vi "Pins Names Read.vi"(4 "error in (no error)":errorcluster, 6 "Container State":T2, 7 "Display State In":T1) -> (0 "error out":errorcluster, 2 "Value":string[](array[string]), 3 "Display State Out":T1)   [LabVIEW 2021, in "roboRIO SPI.xctl"]
uses:
  <vilib>/myRIO/Common/Instrument Driver Framework/Utilities/xctls/roboRIO SPI/roboRIO SPI.xctl
  <vilib>/_xctls/Container State.ctl
  <vilib>/myRIO/Common/Instrument Driver Framework/Utilities/xctls/roboRIO SPI/State.ctl
  <vilib>/_xctls/XControlSupport.lvlib
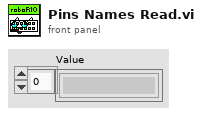
[diagram p1: front panel]
types:
  T1 = typedef "roboRIO SPI.xctl/State.ctl" = cluster{"Pin Disabled?":enum8{"Enabled", "Disabled", "Disabled and Grayed Out"}[], "Pin Name":string[]}
  T2 = typedef "XControlSupport.lvlib/Container State.ctl" = cluster{"Indicator?":bool, "Run Mode?":bool, " Refnum":refnum<vi>}
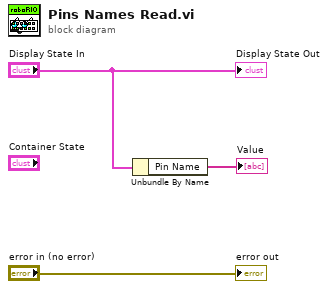
[diagram p0: block diagram]
diagram:
  n1 = Unbundle By Name("Display State In") -> ("Pin Name"=→"Value":string[])
  "error out" <- "error in (no error)"
  "Display State Out" <- "Display State In"
